vi "Connect to TLS Server.vi"() -> ()   [LabVIEW 2023]
doc: "<b>This example, while not specifically written for the LabVIEW Real-Time Module, runs on RT targets.</b>\n\nThis example demonstrates the use of Start TLS to connect to HTTPS webservers, using the OS-provided certificate authority store."
panel:
  in  "Port":u16=443
  in  "Hostname":string="ni.com"
  # "Overview: Demonstrates  connecting to a TLS server and negotiating a TLS connection.\nInstructions:\n1. Set the hostname to that of an HTTPS server (or a server for a protocol which negotiates TLS immediately upon connect).\n2. Change Port if connecting to a protocol other than HTTPS.\n3. Run the VI. TLS will be negotiated over the TCP connection, then the connection is closed."
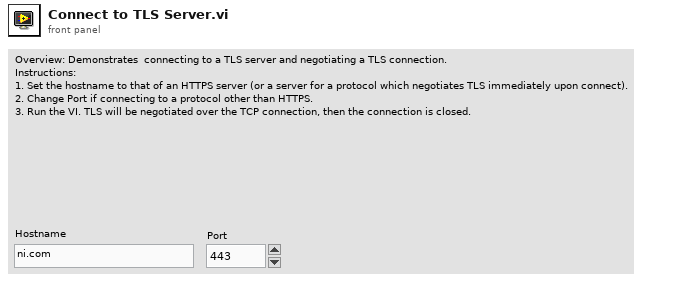
[diagram p1: front panel]
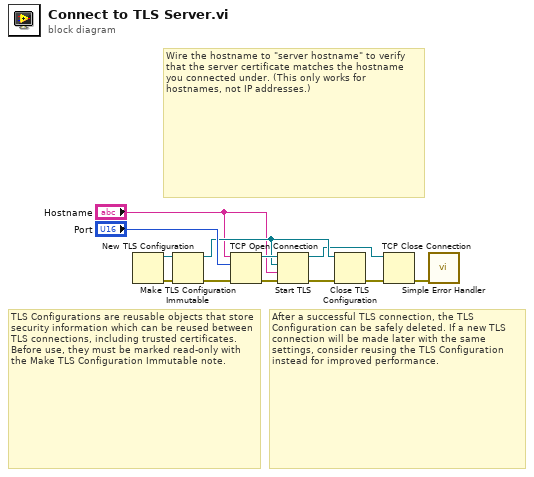
[diagram p0: block diagram]
diagram:
  # "Wire the hostname to \"server hostname\" to verify that the server certificate matches the hostname you connected under. (This only works for hostnames, not IP addresses.)"
  # "TLS Configurations are reusable objects that store security information which can be reused between TLS connections, including trusted certificates. Before use, they must be marked read-only with the Make TLS Configuration Immutable note."
  # "After a successful TLS connection, the TLS Configuration can be safely deleted. If a new TLS connection will be made later with the same settings, consider reusing the TLS Configuration instead for improved performance."
  n1 = New TLS Configuration() -> (0:w9:errorcluster, 3:w10:refnum<k36>)  [unwired: 2 in]
  n2 = Make TLS Configuration Immutable(8:w9, 11:w10) -> (0:w12:errorcluster, 3:w5:refnum<k36>)
  n3 = TCP Open Connection(address="Hostname", remote port or service name="Port", error in (no error)=w12) -> (connection ID=w8:refnum<k5>, error out=w7:errorcluster)  [unwired: 2 in]
  n4 = Start TLS(8:w7, 9:"Hostname", 10:w5, 11:w8) -> (0:w6:errorcluster, 3:w3:refnum<k5>)  [unwired: 2 in, 1 out]
  n5 = Close TLS Configuration(8:w6, 11:w5) -> (0:w4:errorcluster)
  n6 = TCP Close Connection(connection ID=w3, error in (no error)=w4) -> (error out=w1:errorcluster)  [unwired: 1 in, 1 out]
  n7 = call <vilib>:"Simple Error Handler.vi"("error in (no error)"=w1) -> ()  [unwired: 4 in, 5 out]
